vi "Write Data to Excel.vi"(0 "Report In":refnum<class "NI_report.lvclass">, 5 "Header Array":string[](array[string]), 7 "Data Array":string[][](array[string]), 11 "Error In":errorcluster) -> (4 "Report Out":refnum<class "NI_report.lvclass">, 15 "Error Out":errorcluster)   [LabVIEW 2023]
uses:
  <vilib>/Utility/NIReport.llb/NI_report.lvclass
  <vilib>/addons/_office/_exclsub.llb/font.ctl
  <vilib>/addons/_office/excel.llb/Excel Easy Table (str).vi
  <vilib>/addons/_office/NI_ReportGenerationToolkit.lvlib
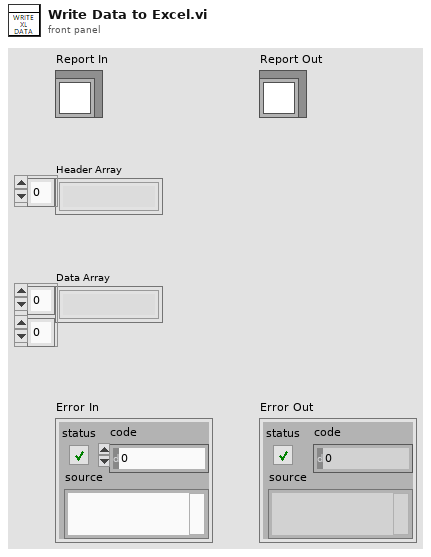
[diagram p1: front panel]
types:
  T1 = typedef "NI_ReportGenerationToolkit.lvlib/font.ctl" = cluster{"font name":string, "font size":dbl, "bold":u16, "italic":u16, "underline":u16, "strike through":u16, "font color":u32}
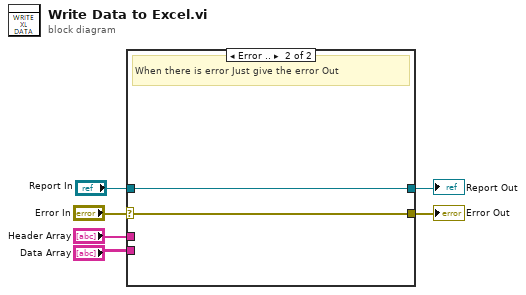
[diagram p0: block diagram]
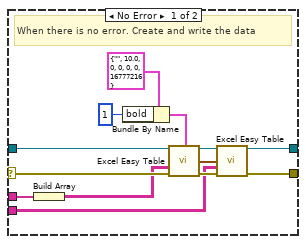
[diagram p2: hidden frame]
diagram:
  n1 = case shown="Error .." "Error In" {
    selector: "Error In" -> [w13 w21]
    tunnel: [w9 w21] -> w6
    tunnel: "Header Array" -> [w12 _]
    tunnel: "Data Array" -> [w11 _]
    tunnel: "Report In" -> [w8 w20]
    tunnel: [w7 w20] -> w2
    frame No Error {
      # "When there is no error. Create and write the data"
      n2 = Build Array(w12) -> (w10:string[][])
      n3 = Bundle By Name(cluster=T1 {"font name"="", "font size"=10.0, "bold"=0, "italic"=0, "underline"=0, "strike through"=0, "font color"=16777216} ("font"), "bold"=u16 1) -> (w18:T1)
      n4 = call-poly <vilib>:"Excel Easy Table.vi"("report in"=w8, "font"=w18, "text data"=w10, "error in (no error)"=w13) -> ("report out"=w14:refnum<class "NI_report.lvclass">, "next cell bottom-left"=w19:cluster{"row":i32, "column":i32}, "error out"=w15:errorcluster)  [unwired: 7 in, 2 out]
      n5 = call-poly <vilib>:"Excel Easy Table.vi"("report in"=w14, "start (0, 0)"=w19, "text data"=w11, "error in (no error)"=w15) -> ("report out"=w7:refnum<class "NI_report.lvclass">, "error out"=w9:errorcluster)  [unwired: 7 in, 3 out]
    }
    frame Error {
      # "When there is error Just give the error Out"
    }
  }
  "Error Out" <- w6
  "Report Out" <- w2
